vi "MassData Parameter Support Demo 2.vi"() -> ()   [LabVIEW 2017]
uses:
  MassData-Parameter/_support/Operation-FGV-MassData.ctl
  b1bc9acf-e850-46c1-b3cf-cc66e9187574.vi
  537af5e7-dcec-4c12-9422-676432e19088.vi
  MassData-Parameter/CSM MassData Parameter Support.lvlib
panel:
  in  "stop":bool
  out "Thermometer":cluster{dbl, dbl}(slide)={0.0, 6224.489795918367} scale=0.0..1000000.0 scale format="%#_6p"
  out "Argument":string
  out "Waveform Graph":waveform(dbl)(graph)
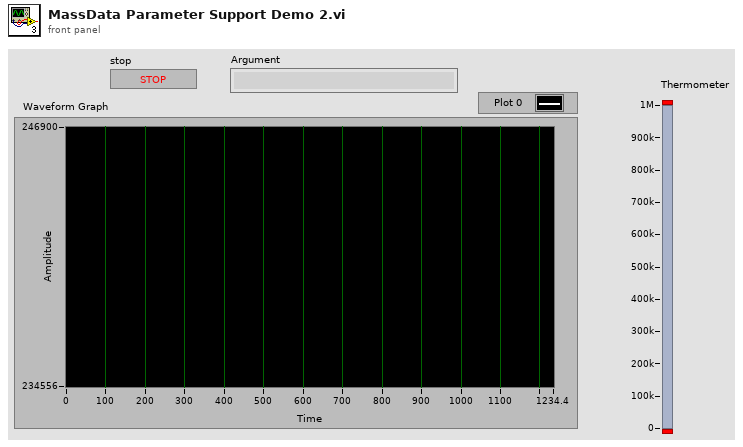
[diagram p1: front panel]
types:
  T1 = typedef "CSM MassData Parameter Support.lvlib/Operation-FGV-MassData.ctl" = enum16{"Initialize", "Read", "Write", "Status", "Release"}
  T2 = typedef "CSM MassData Parameter Support.lvlib/Def-MassDataOper-Status.ctl" = cluster{"Start":i32, "Size":i32, "Total":i32}
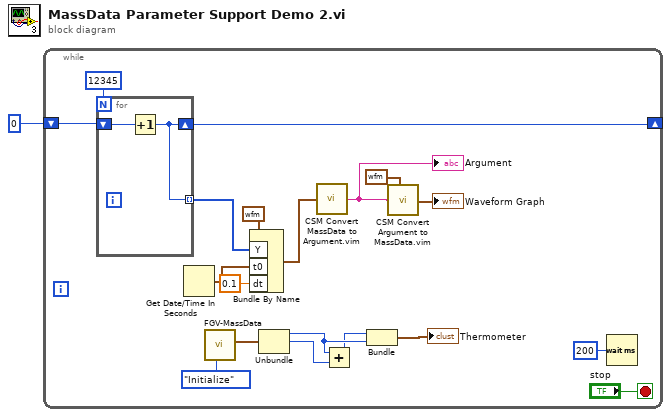
[diagram p0: block diagram]
diagram:
  n1 = while {
    shift-right: [w9] -> _
    shift-left: 0 -> [w10]
    stop <- "stop" stop-if-true
    n2 = for {
      N: 12345 -> [_]
      tunnel: [w21] -> w4 mode=indexing
      shift-right: [w21] -> w9
      shift-left: w10 -> [w22]
      n3 = Increment(x=w22) -> (x+1=w21:i32)
    }
    n4 = Get Date/Time In Seconds() -> (seconds since 1Jan1904=w6:timestamp)
    n5 = call "FGV-MassData.vi"("Operation"=Operation-FGV-MassData."Initialize") -> ("Active Write Oper"=w13:T2)  [unwired: 7 in, 3 out]
    n6 = Bundle By Name(cluster=waveform(dbl) {"t0"=timestamp(0 s since 1904-01-01), "dt"=1.0, "Y"=[]} ("Waveform"), "Y"=w4, "t0"=w6, "dt"=0.1) -> (w3:waveform(dbl))
    n7 = Unbundle(w13) -> ("Start"=w16:i32, "Size"=w14:i32)  [unwired: 1 out]
    n8 = call "CSM Convert MassData to Argument.vim"("DBL"=w3) -> ("Argument"=w8:string)  [unwired: 8 in]
    "Argument" <- w8
    n9 = Add(x=w16, y=w14) -> (x+y=w15:i32)
    n10 = Bundle(w15, "Start"=w16) -> (→"Thermometer":cluster{i32, "Start":i32})  [unwired: 1 in]
    n11 = call "CSM Convert Argument to MassData.vim"("Type"=waveform(dbl) {"t0"=timestamp(0 s since 1904-01-01), "dt"=1.0, "Y"=[]} ("Waveform"), "HEX Argument"=w8) -> ("DBL"=→"Waveform Graph":waveform(dbl))  [unwired: 7 in]
    n12 = Wait (ms)(milliseconds to wait=u32 200) -> ()  [unwired: 1 out]
  }
